vi "Demo_Andon_logic.vi"(9 "Inputs past":bool[](array[boolean]), 10 "Inputs":bool[](array[boolean]), 11 "Outputs past":bool[](array[boolean])) -> (1 "Inputs to save":bool[](array[boolean]), 2 "Outputs OUT":bool[](array[boolean]), 6 "Outputs to card":string[](array[string]))   [LabVIEW 2017]
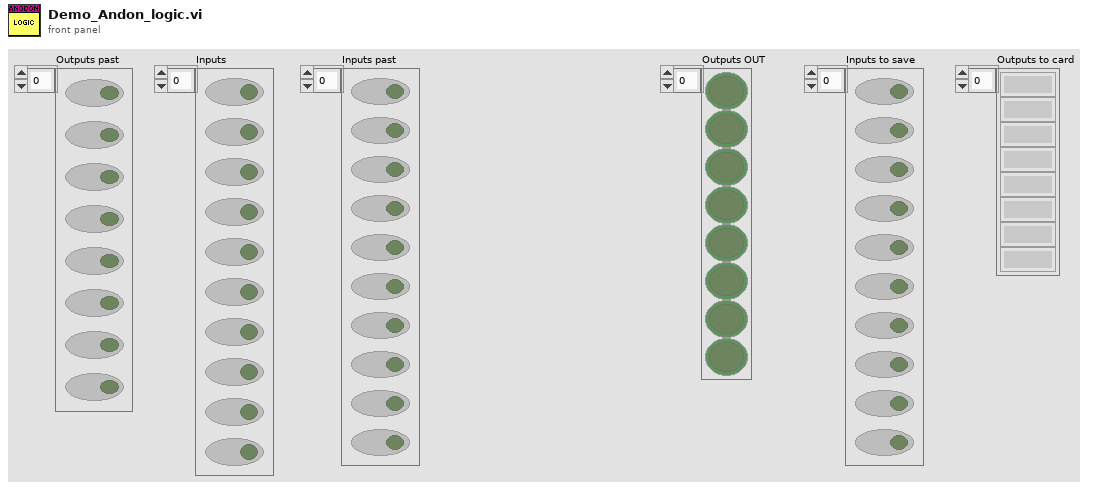
[diagram p1: front panel]
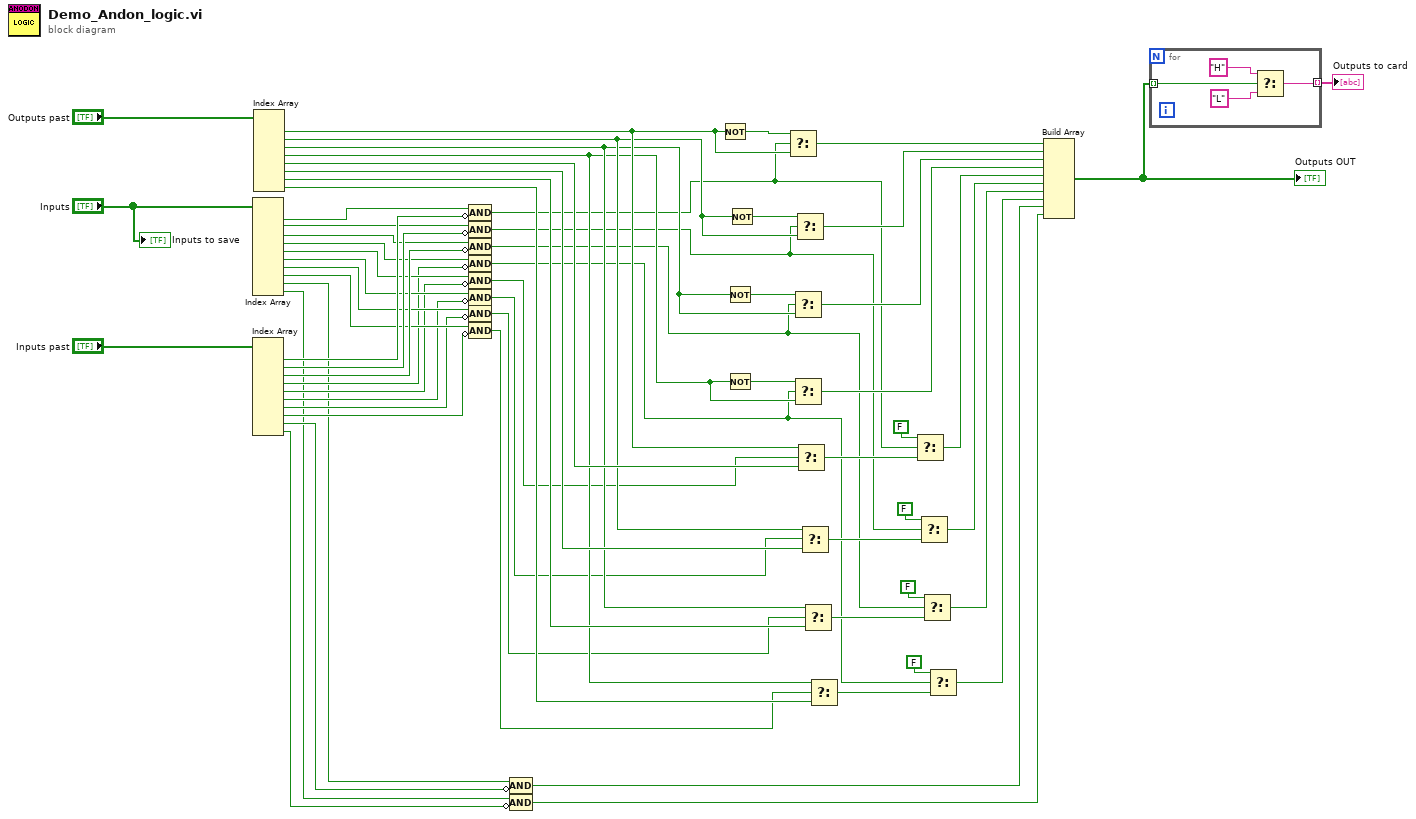
[diagram p0: block diagram]
diagram:
  n1 = Index Array(array="Inputs") -> (element #1=w31:bool, element #2=w29:bool, element #3=w25:bool, element #4=w23:bool, element #5=w22:bool, element #6=w21:bool, element #7=w20:bool, element #8=w19:bool, element #9=w3:bool, element #10=w4:bool)  [unwired: 10 in]
  n2 = Index Array(array="Inputs past") -> (element #1=w30:bool, element #2=w28:bool, element #3=w24:bool, element #4=w18:bool, element #5=w17:bool, element #6=w16:bool, element #7=w15:bool, element #8=w14:bool, element #9=w5:bool, element #10=w6:bool)  [unwired: 10 in]
  n3 = Index Array(array="Outputs past") -> (element #1=w52:bool, element #2=w48:bool, element #3=w44:bool, element #4=w40:bool, element #5=w55:bool, element #6=w49:bool, element #7=w45:bool, element #8=w41:bool)  [unwired: 8 in]
  n4 = Compound Arithmetic op=AND(w31, invert w30) -> (w27:bool)
  n5 = Compound Arithmetic op=AND(w29, invert w28) -> (w26:bool)
  n6 = Compound Arithmetic op=AND(w25, invert w24) -> (w13:bool)
  n7 = Compound Arithmetic op=AND(w23, invert w18) -> (w12:bool)
  n8 = Compound Arithmetic op=AND(w22, invert w17) -> (w11:bool)
  n9 = Compound Arithmetic op=AND(w21, invert w16) -> (w10:bool)
  n10 = Compound Arithmetic op=AND(w20, invert w15) -> (w9:bool)
  n11 = Compound Arithmetic op=AND(w19, invert w14) -> (w8:bool)
  n12 = Compound Arithmetic op=AND(w3, invert w5) -> (w2:bool)
  n13 = Compound Arithmetic op=AND(w4, invert w6) -> (w1:bool)
  n14 = Not(x=w52) -> (.not. x?=w58:bool)
  n15 = Not(x=w44) -> (.not. x?=w57:bool)
  n16 = Not(x=w40) -> (.not. x?=w56:bool)
  n17 = Not(x=w48) -> (.not. x?=w59:bool)
  n18 = Select(t=w58, s=w27, f=w52) -> (s? t:f=w39:bool)
  n19 = Select(t=w57, s=w13, f=w44) -> (s? t:f=w37:bool)
  n20 = Select(t=w56, s=w12, f=w40) -> (s? t:f=w36:bool)
  n21 = Select(t=w59, s=w26, f=w48) -> (s? t:f=w38:bool)
  n22 = Select(t=w52, s=w11, f=w55) -> (s? t:f=w54:bool)
  n23 = Select(t=w48, s=w10, f=w49) -> (s? t:f=w51:bool)
  n24 = Select(t=w44, s=w9, f=w45) -> (s? t:f=w46:bool)
  n25 = Select(t=w40, s=w8, f=w41) -> (s? t:f=w43:bool)
  n26 = Select(t=FALSE ("Rising Edge"), s=w27, f=w54) -> (s? t:f=w35:bool)
  n27 = Select(t=FALSE ("Rising Edge"), s=w26, f=w51) -> (s? t:f=w34:bool)
  n28 = Select(t=FALSE ("Rising Edge"), s=w13, f=w46) -> (s? t:f=w33:bool)
  n29 = Select(t=FALSE ("Rising Edge"), s=w12, f=w43) -> (s? t:f=w32:bool)
  n30 = Build Array(w39, w38, w37, w36, w35, w34, w33, w32, w2, w1) -> (w63:bool[])
  "Outputs OUT" <- w63
  n31 = for {
    tunnel: w63 -> [w65] mode=indexing
    tunnel: [w64] -> w62 mode=indexing
    n32 = Select(t="H", s=w65, f="L") -> (s? t:f=w64:string)
  }
  "Outputs to card" <- w62
  "Inputs to save" <- "Inputs"
